vi "Add Recipe Rev1.vi"(4 "Temperature":u16, 5 "Speed":u16, 8 "error in (no error)":errorcluster, 10 "Time Limit":u16, 11 "MASTER in":refnum<class "MASTER.lvclass">) -> (0 "error out":errorcluster, 3 "MASTER out":refnum<class "MASTER.lvclass">)   [LabVIEW 2014, in "Files Library.lvlib" / "MASTER.lvclass"]
uses:
  MASTER.lvclass
  CONTROL/Recipes Indicators.ctl
  MASTER.lvclass/MASTER.ctl
  Files Library.lvlib
panel:
  in  "new element/subarray":T1
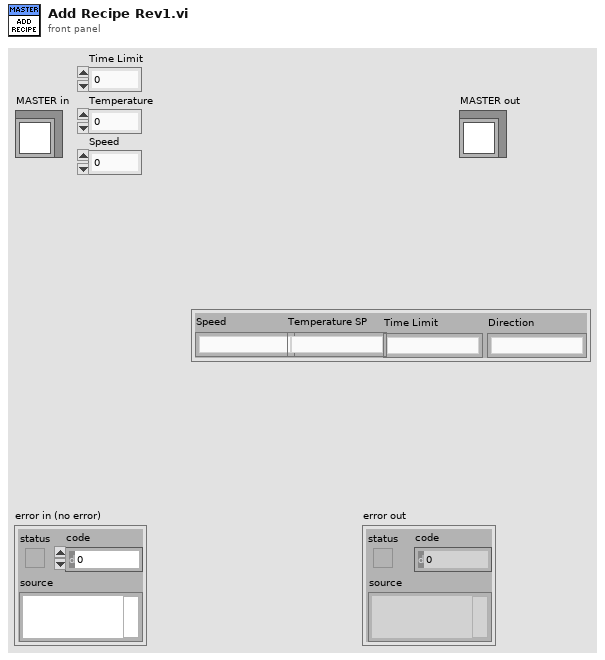
[diagram p1: front panel]
types:
  T1 = typedef "Recipes Indicators.ctl" = cluster{"Speed":string, "Temperature SP":string, "Time Limit":string, "Direction":string}
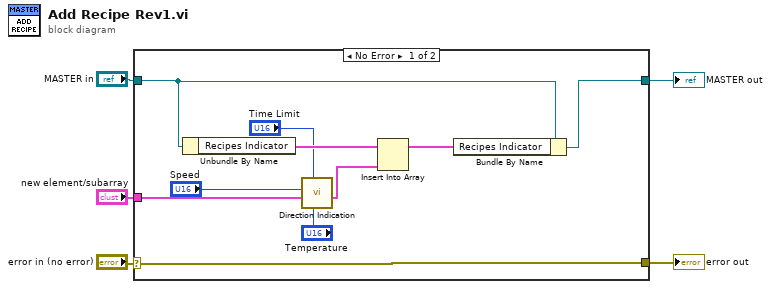
[diagram p0: block diagram]
diagram:
  n1 = case shown="No Error" "error in (no error)" {
    selector: "error in (no error)" -> [w15 w17]
    tunnel: [w15 w17] -> w4
    tunnel: [w13 w16] -> w2
    tunnel: "MASTER in" -> [w14 w16]
    tunnel: "new element/subarray" -> [w9 _]
    frame No Error {
      n2 = Unbundle By Name(w14) -> ("Recipes Indicator"=w12:T1[])
      n3 = call "Direction Indication.vi"("Temperature"="Temperature", "Time Limit"="Time Limit", "new element/subarray 2"=w9, "Speed"="Speed") -> ("new element/subarray 3"=w10:T1)  [unwired: 7 in]
      n4 = Insert Into Array(array=w12, new element=w10) -> (w11:T1[])  [unwired: 1 in]
      n5 = Bundle By Name(cluster=w14, "Recipes Indicator"=w11) -> (w13:refnum<class "MASTER.lvclass">)
    }
    frame Error {
    }
  }
  "error out" <- w4
  "MASTER out" <- w2
